vi "commit VI reference.vi"(8 "error in":errorcluster, 10 "VI Refnum":refnum<vi>, 11 "UI Reference configuration in":refnum<class "UI Reference configuration.lvclass">) -> (0 "error out":errorcluster, 3 "UI Reference configuration out":refnum<class "UI Reference configuration.lvclass">)   [LabVIEW 2013, in "UI Reference configuration.lvclass"]
uses:
  UI Reference configuration.lvclass
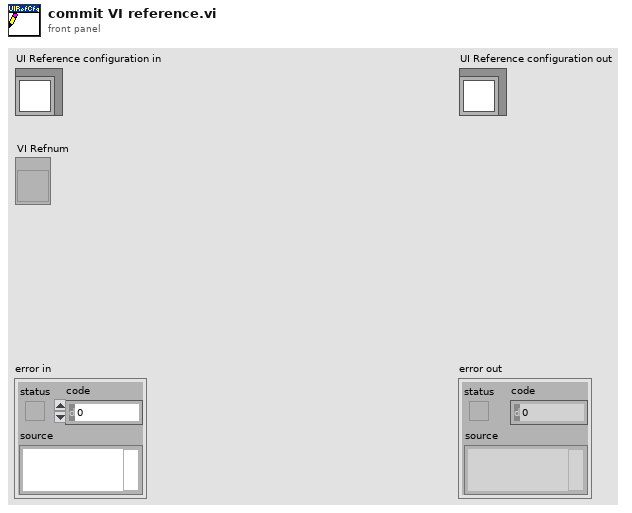
[diagram p1: front panel]
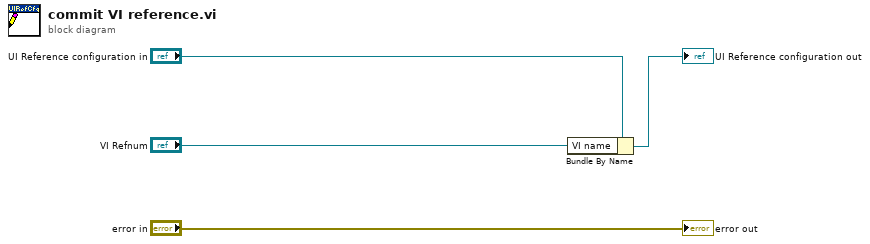
[diagram p0: block diagram]
diagram:
  n1 = Bundle By Name(cluster="UI Reference configuration in", "VI name"="VI Refnum") -> (→"UI Reference configuration out":refnum<class "UI Reference configuration.lvclass">)
  "error out" <- "error in"
